vi "SignalGenerator.vi"(10 "phase":fxp<+,64,64>, 11 "Reset":bool) -> (0 "data_valid":bool, 1 "Cos":fxp<+/-,16,0>, 2 "Sin":fxp<+/-,16,0>)   [LabVIEW 2013]
uses:
  <vilib>/rvi/IPIntegrationNode/IPINode_Utilities/niFpgaIPINodeSimCore.vi
  <vilib>/rvi/FXPMathLib/FxpInterpret/XNode/nifxpmath_Interpret.xnode
  <vilib>/rvi/XilinxIP/XIPIN_XNode/niFpgaXIPIN.xnode
  DDS_1/DDS Compiler/DDS_Compiler_AEE5C67338364F1EA41DEF5F1D6503D7.dll
  <vilib>/rvi/IPIntegrationNode/IPINode_Xnode/niFpgaIPINode.xnode
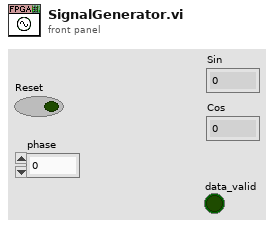
[diagram p1: front panel]
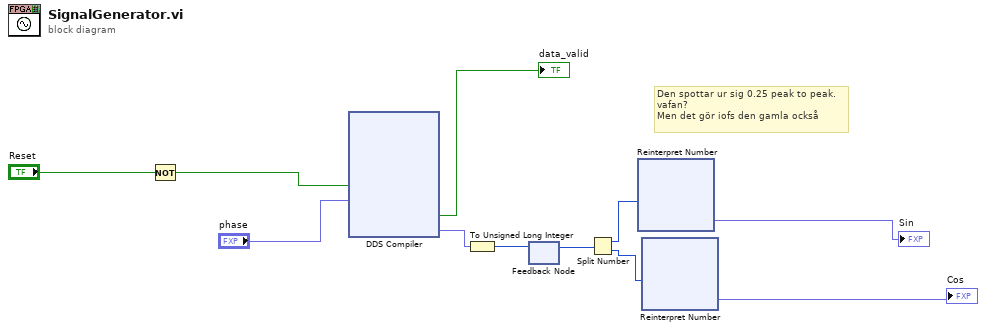
[diagram p0: block diagram]
diagram:
  # "Den spottar ur sig 0.25 peak to peak.\nvafan?\nMen det gör iofs den gamla också"
  n1 = Not(x="Reset") -> (.not. x?=w3:bool)
  n2 = xnode ("DDS Compiler")("aresetn"=w3, "s_axis_phase_tdata"="phase") -> ("m_axis_data_tvalid"=→"data_valid":bool, "m_axis_data_tdata"=w7:fxp<+,32,32>)  [unwired: 2 in]
  n3 = To Unsigned Long Integer(number=w7) -> (unsigned 32bit integer=w2:u32)
  n4 = feedback #1() -> (w1:u32)  [unwired: 1 in]
  n5 = feedback-in #1(w2) -> ()
  n6 = Split Number(x=w1) -> (hi(x)=w9:u16, lo(x)=w8:u16)
  n7 = xnode "Reinterpret Number"("x"=w9) -> ("y"=→"Sin":fxp<+/-,16,0>)
  n8 = xnode "Reinterpret Number"("x"=w8) -> ("y"=→"Cos":fxp<+/-,16,0>)
